vi "Disable Alarm on NaN.vi"(11 "numeric alarm settings in":T1={"enable? (F)"=FALSE, "name"="", "alarm type"=enum."LO_LO", "level/change"=nan, "deadband/time"=nan, "alarm delay"=0.0, "priority"=0, "ack type"=enum."Auto", "area"="", "description"="", "log? (T)"=FALSE}) -> (3 "numeric alarm settings out":T1={"enable? (F)"=FALSE, "name"="", "alarm type"=enum."LO_LO", "level/change"=nan, "deadband/time"=nan, "alarm delay"=0.0, "priority"=0, "ack type"=enum."Auto", "area"="", "description"="", "log? (T)"=FALSE})   [LabVIEW 2018, in "Dynamic Shared Variables.lvlib"]
doc: "If level of the alarm is NaN, then disable the alarm."
uses:
  Dynamic Shared Variables.lvlib
  Tag VIs/Numeric Alarm Settings Cluster.ctl
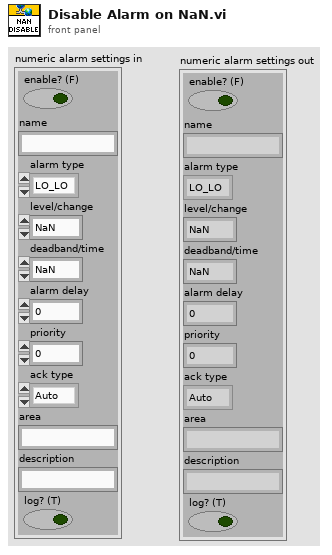
[diagram p1: front panel]
types:
  T1 = typedef "Numeric Alarm Settings Cluster.ctl" = cluster{"enable? (F)":bool, "name":string, "alarm type":enum16{"HI_HI", "HI", "LO", "LO_LO"}, "level/change":dbl, "deadband/time":dbl, "alarm delay":dbl, "priority":u32, "ack type":enum16{"Auto", "User", "None", "Each Occurrence"}, "area":string, "description":string, "log? (T)":bool}
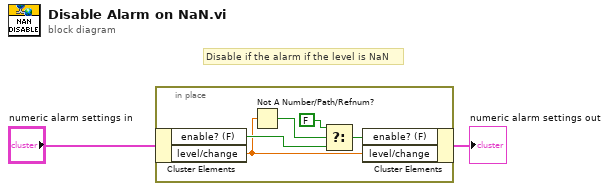
[diagram p0: block diagram]
diagram:
  # "Disable if the alarm if the level is NaN"
  n1 = in-place {
    n2 = in-place-cluster #1("numeric alarm settings in") -> ("enable? (F)"=w4:bool, "level/change"=w3:dbl)
    n3 = Not A Number/Path/Refnum?(number/path/refnum=w3) -> (NaN/Path/Refnum?=w7:bool)
    n4 = Select(t=FALSE, s=w7, f=w4) -> (s? t:f=w5:bool)
    n5 = in-place-cluster #1("enable? (F)"=w5, "level/change"=w3) -> (→"numeric alarm settings out":T1)
  }
